vi "licore (main).vi"(5 "Licor-parameter":refnum<vi>, 7 "manual control":refnum<vi>, 8 "raw data":refnum<vi>, 9 "VISA resource name":refnum<visa-resource-name>="ASRL1::INSTR" caption="VISA-Ressourcenname", 10 "Licor-parameter":T1={"CO2 ref"=392.0, "CO2 span"=402.0, "H2O ref"=0.0, "H2O span"=0.0, "Zi"=1.2, "Zt"=0.0, "Zm"=0.0, "S"=1.0, "Temp [C]"=50.0, "Pressure [hPa]"=135.0, "Licor-Sources"=["CO2A W", "CO2B W", "H2OA W", "H2OB W", "T C", "T V", "P kPa", "P V", "RH %", "CO2A um/m", "CO2B um/m", "H2OA mm/m", "H2OB mm/m"], "Licor-Pump"="Off", "Zeitstempel"=timestamp(0 s since 1904-01-01)} {"Pressure [hPa]" format="%.2g"; "Temp [C]" format="%.2f"; "CO2 ref" format="%.2f"; "CO2 span" format="%.2g"; "H2O ref" format="%.2g"; "H2O span" format="%.2g"}, 11 "graph":refnum<vi>) -> ()   [LabVIEW 2010]
uses:
  control/Licor-Parameter.ctl
  Licor-Steuerung/LicorLI7000/conventions/Licor-Source.ctl
  control/Licor-Pump.ctl
  <vilib>/Platform/TimedLoop/XDataNode/nitl_modes.ctl
  <vilib>/Platform/TimedLoop/XDataNode/XDataNode.xnode
  <vilib>/Platform/TimedLoop/XDataNode/timing_clust.ctl
  <vilib>/Platform/TimedLoop/XDataNode/wakeup.ctl
  control/Licor-Sequences.ctl
  <vilib>/Instr/_visa.llb/VISA Configure Serial Port (Instr).vi
  <vilib>/Platform/TimedLoop/XDataNode/XDNodeRunTimeDep.lvlib
  Licor-Steuerung/LicorLI7000/LicorLI7000.lvlib
panel:
  out "Licor-parameter out":T1={"CO2 ref"=0.0, "CO2 span"=0.0, "H2O ref"=0.0, "H2O span"=0.0, "Zi"=0.0, "Zt"=0.0, "Zm"=0.0, "S"=0.0, "Temp [C]"=50.0, "Pressure [hPa]"=135.0, "Licor-Sources"=["CO2A W", "CO2B W", "H2OA W", "H2OB W", "T C", "T V", "P kPa", "P V", "RH %", "CO2A um/m", "CO2B um/m", "H2OA mm/m", "H2OB mm/m"], "Licor-Pump"="Off", "Zeitstempel"=timestamp(0 s since 1904-01-01)} {"Pressure [hPa]" format="%.2g"; "Temp [C]" format="%.2f"; "CO2 ref" format="%.2f"; "CO2 span" format="%.2g"; "H2O ref" format="%.2g"; "H2O span" format="%.2g"}
  out "graph":cluster{"X":dbl[], "Y":dbl[]}(graph)
  out "graph":cluster{"time (cRio)":dbl[], "data":dbl[]}[](array[cluster])
  out "time":i64
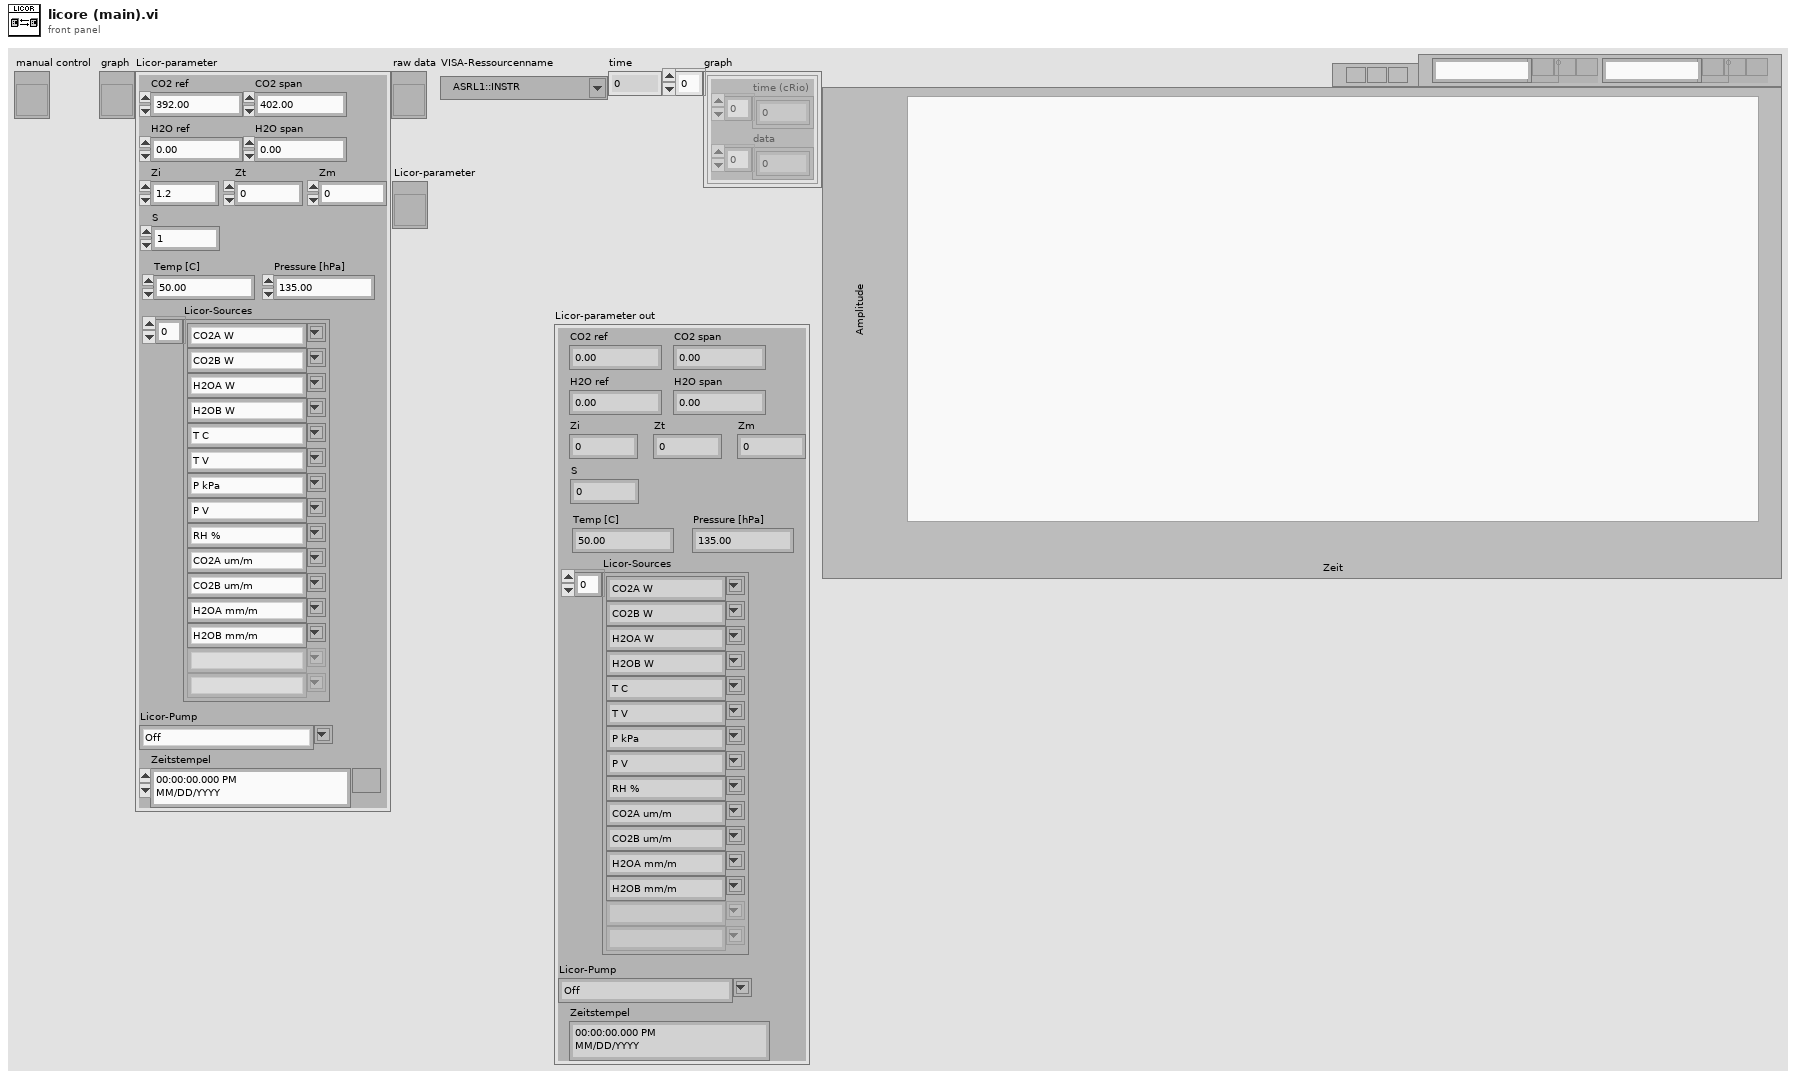
[diagram p1: front panel]
types:
  T1 = typedef "Licor-Parameter.ctl" = cluster{"CO2 ref":dbl, "CO2 span":dbl, "H2O ref":dbl, "H2O span":dbl, "Zi":dbl, "Zt":dbl, "Zm":dbl, "S":dbl, "Temp [C]":dbl, "Pressure [hPa]":dbl, "Licor-Sources":T2[], "Licor-Pump":T3, "Zeitstempel":timestamp}
  T2 = typedef "LicorLI7000.lvlib/Licor-Source.ctl" = string
  T3 = typedef "Licor-Pump.ctl" = string
  T4 = typedef "Licor-Sequences.ctl" = enum16{"test", "WAIT", "warmup", "initialize", "calibrate Z", "calibrate S"}
  T5 = typedef "XDNodeRunTimeDep.lvlib/nitl_modes.ctl" = enum32{"No Change", "Process missed periods, maintain original phase", "Discard missed periods, maintain original phase", "Process missed periods, ignore original phase", "Discard missed periods, ignore original phase"}
  T6 = typedef "XDNodeRunTimeDep.lvlib/timing_clust.ctl" = cluster{"Expected End [f-1]":u64, "Actual End [f-1]":u64, "Finished Late? [f-1]":bool, "Expected End [i-1]":u64, "Actual End [i-1]":u64, "Finished Late? [i-1]":bool, "Expected Start [i]":u64, "Actual Start [i]":u64, "Expected Start [f]":u64, "Actual Start [f]":u64, "Source Name":string, "Structure Name":string, "Period":i64, "Deadline":i64, "Offset":i64, "Start":i64, "Priority":i32, "Timeout":i32, "Mode":T5, "Wakeup Reason":T7, "Error":errorcluster, "Source Type":string, "Secondary Source Type":string, "Global End Time":u64, "Global Start Time":u64, "Frame Duration":u64, "Iteration Duration":u64, "Assigned CPU":i32, "I/O Scan Engine Mode":u32}
  T7 = typedef "XDNodeRunTimeDep.lvlib/wakeup.ctl" = enum32{"Normal", "Aborted", "Asynchronous wakeup", "Timing source error", "Timed loop error", "Timeout"}
  T8 = typedef "VI-data Save.ctl" = cluster{"Dateipfad save data":path, "file ref":refnum<file>, "number":i64, "Period [s]":i64, "Fehler (Ausgang)":errorcluster}
  T9 = cluster{"sequence manual":T4, "sequence manual ?":bool}
  T10 = cluster{"time (global)":dbl, "MPV":i32, "manual control":cluster{"sequence manual":T4, "sequence manual ?":bool}}
  T11 = cluster{"sequence":T4, "time (next command)":dbl}
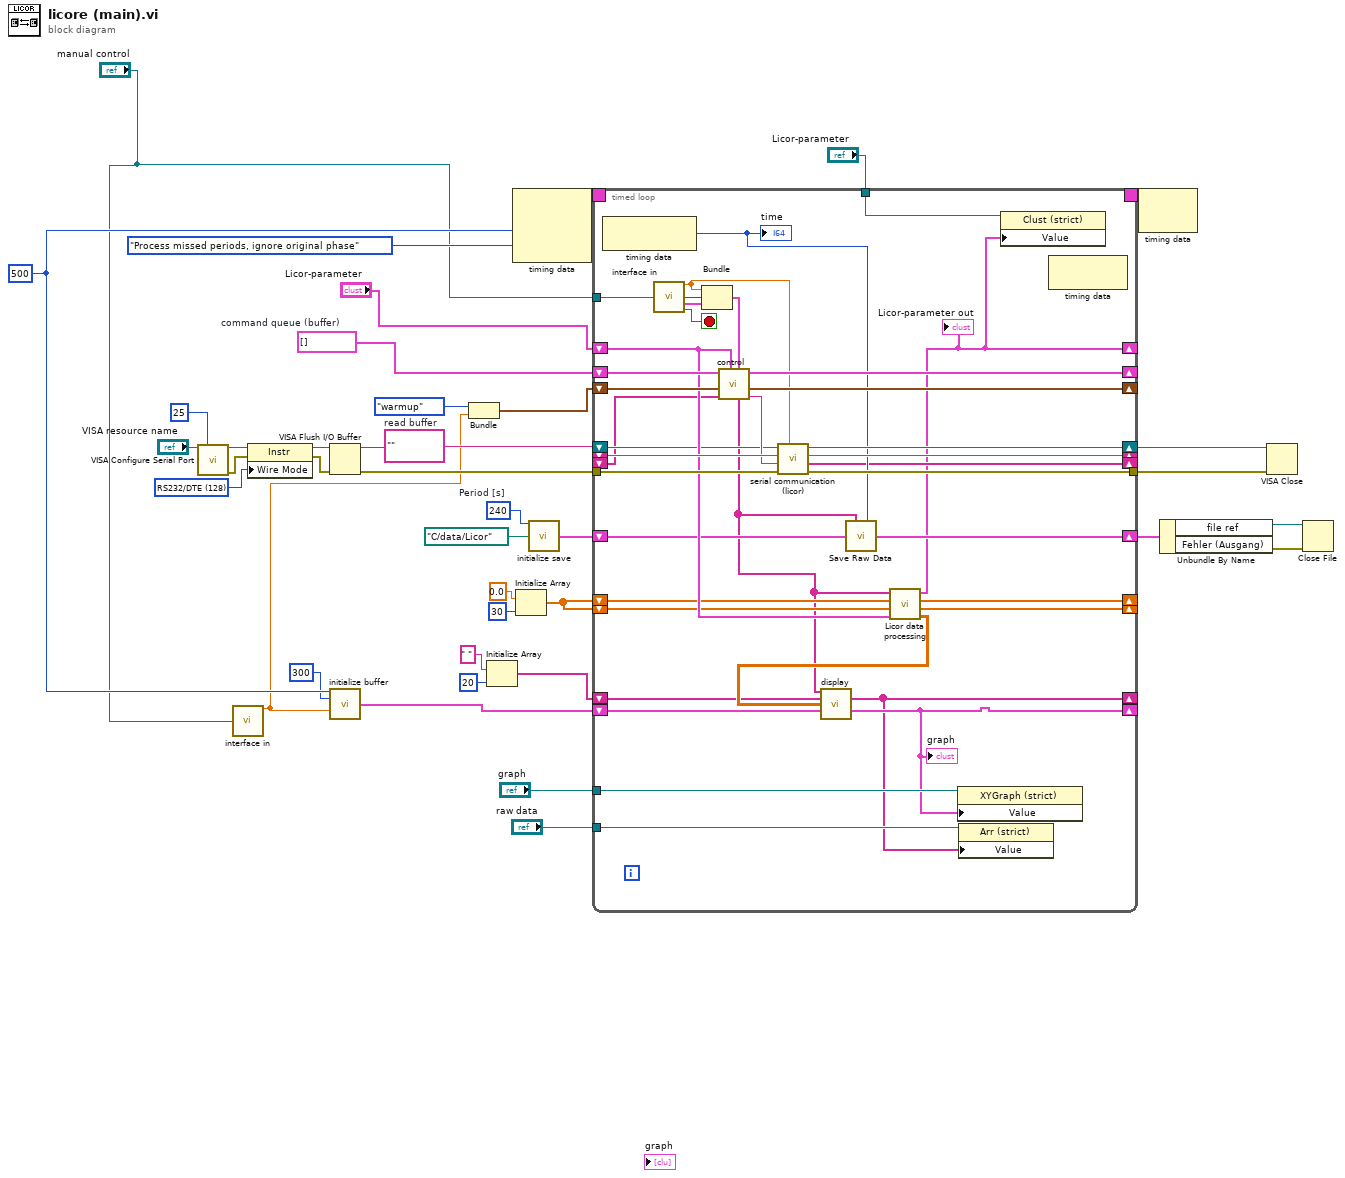
[diagram p0: block diagram]
diagram:
  w11 = i64 240  # Period [s]
  w24 = cluster{"Zeit [s]":i32, "Befehl":string}[] []  # command queue (buffer)
  w28 = ""  # read buffer
  w31 = i16 128 items=["Unknown"=-1, "RS485/Wire4"=0, "RS485/Wire2-EchoDTR"=1, "RS485/Wire2-CtrlDTR"=2, "RS485/Wire2-Auto"=3, "RS232/DTE"=128, "RS232/DCE"=129, "RS232/AUTO"=130] ("Serial Settings:Wire Mode")
  w27 = i64 500 ("Periode")
  n1 = call-poly "VISA Configure Serial Port"("VISA resource name"="VISA resource name", "timeout (10sec)"=u32 25) -> ("VISA resource name out"=w35:refnum<visa-resource-name>, "error out"=w34:errorcluster)  [unwired: 12 in]
  n2 = call "interface in.vi"("manual control"="manual control") -> ("time (global)"=w23:dbl)  [unwired: 11 in, 3 out]
  n3 = property class="Instr"(reference=w35, error in=w34, "Wire Mode"=w31) -> (reference out=w33:refnum<visa-resource-name>, error out=w32:errorcluster)
  n4 = VISA Flush I/O Buffer(VISA resource name=w33, error in (no error)=w32) -> (VISA resource name out=w12:refnum<visa-resource-name>, error out=w29:errorcluster)  [unwired: 1 in]
  n5 = call "initialize buffer.vi"("Periode"=w27, "samplesize plots"=i64 300, "initial time"=w23) -> ("buffer plot"=w6:cluster{"X":dbl[], "Y":dbl[]})  [unwired: 12 in]
  n6 = Bundle(Licor-Sequences."warmup", "time (global)"=w23) -> (w21:cluster{T4, "time (global)":dbl})  [unwired: 1 in]
  n7 = Initialize Array(" ", 20 ("Dimension")) -> (w18:string[])
  n8 = node-c288(w27, nitl_modes."Process missed periods, ignore original phase" ("Modus")) -> (w39:T6)  [unwired: 1 in]
  n9 = Initialize Array(0.0 ("time (globale Variable)"), 30 ("Dimension")) -> (w2:dbl[])
  n10 = call "initialize save.vi"("Period [s]"=w11, "cRio data path"=path "C:/data/Licor") -> ("VI-data Save"=w13:T8)  [unwired: 13 in]
  n11 = timed-loop {
    timing: w39 -> [_]
    timing-out: [_] -> w38
    tunnel: w29 -> [w76]
    shift-right: [w64] -> _
    shift-left: w28 -> [w75]
    shift-right: [w57] -> w26
    shift-left: w12 -> [w58]
    tunnel: [w74] -> w25
    shift-right: [w43] -> _
    shift-left: w6 -> [w46]
    shift-right: [w72] -> _
    shift-left: w24 -> [w71]
    shift-right: [w70] -> _
    shift-left: w21 -> [w63]
    shift-right: [w55] -> w10
    shift-left: w13 -> [w56]
    tunnel: "graph" -> [w65]
    shift-right: [w40] -> _
    shift-left: "Licor-parameter" -> [w59]
    shift-right: [w42] -> _
    shift-left: w18 -> [w45]
    tunnel: "raw data" -> [w61]
    tunnel: "manual control" -> [w60]
    shift-right: [w51] -> _
    shift-left: w2 -> [w48]
    shift-right: [w53] -> _
    shift-left: _ -> [w52]
    shift-right: [w50] -> _
    shift-left: w2 -> [w49]
    tunnel: "Licor-parameter" -> [w41]
    stop <- w68 stop-if-true
    n12 = node-c288() -> (w54:i64)  [unwired: 1 in]
    "time" <- w54
    n13 = call "interface in.vi"("manual control"=w60) -> ("time (global)"=w62:dbl, "MPV"=w69:i32, "manual control"=w67:T9, "global stop"=w68:bool)  [unwired: 11 in]
    n14 = Bundle("time (global)"=w62, "MPV"=w69, "manual control"=w67) -> (w66:T10)  [unwired: 1 in]
    n15 = call "control.vi"("control"=w66, "command parameter"=w59, "Licor-output"=w52, "sequence in"=w63, "command queue in"=w71) -> ("Licor command"=w73:string, "sequence out"=w70:T11, "command queue out"=w72:cluster{"Zeit [s]":i32, "Befehl":string}[], "data"=w44:string[])  [unwired: 3 in]
    n16 = call "serial communication (licor).vi"("time (global)"=w62, "Fehler"=w76, "command"=w73, "read buffer in"=w75, "VISA resource out"=w58) -> ("Fehler (Ausgang)"=w74:errorcluster, "Licor-output"=w53:string[], "read buffer out"=w64:string, "VISA resource out 2"=w57:refnum<visa-resource-name>)
    n17 = call "Save Raw Data.vi"("data"=w44, "time [ms]"=w54, "VI-data Save"=w56) -> ("VI-data Save out"=w55:T8)  [unwired: 12 in]
    n18 = call "Licor data processing.vi"("command parameter"=w59, "mittel CO2B W"=w48, "mittel CO2A W"=w49, "raw data"=w44) -> ("time; CO2 data"=w47:dbl[][], "mittel CO2B W out"=w51:dbl[], "mittel CO2A W out"=w50:dbl[], "command parameter"=w40:T1)  [unwired: 4 in]
    "Licor-parameter out" <- w40
    n19 = call "display.vi"("raw data"=w44, "raw data buffer"=w45, "measurement data"=w47, "buffer plot"=w46) -> ("raw data buffer out"=w42:string[], "buffer plot out"=w43:cluster{"X":dbl[], "Y":dbl[]})  [unwired: 10 in]
    "graph" <- w43
    n20 = property on="Eigenschaftsknoten" class="XYGraph (strict)"(reference=w65, "Value"=w43) -> ()  [unwired: 1 in, 2 out]
    n21 = property on="Eigenschaftsknoten" class="Arr (strict)"(reference=w61, "Value"=w42) -> ()  [unwired: 1 in, 2 out]
    n22 = property class="Clust (strict)"(reference=w41, "Value"=w40) -> ()  [unwired: 1 in, 2 out]
    n23 = node-c288() -> ()  [unwired: 1 in, 1 out]
  }
  n24 = node-c288(w38) -> ()  [unwired: 1 out]
  n25 = Unbundle By Name(w10) -> ("file ref"=w9:refnum<file>, "Fehler (Ausgang)"=w8:errorcluster)
  n26 = VISA Close(VISA resource name=w26, error in (no error)=w25) -> ()  [unwired: 1 out]
  n27 = Close File(refnum=w9, error in=w8) -> ()  [unwired: 2 out]
